vi "color2resistance.vi"() -> (5 "finish":bool, 6 "Correct or not":bool, 7 "Answear Time (sec)":dbl)   [LabVIEW 2014]
panel:
  out "Final Ans":dbl
  out "Band 3":u32(colorbox)=16750592
  out "Band 2":u32(colorbox)=16067327
  out "Band 1":u32(colorbox)=16776960
  in  "Resistor Colors":u32[](array[colorbox])=[0, 16730368, 16711680, 16750592, 16776960, 6618880, 3381759, 16067327, 11776947, 16448250]
  out "Question":dbl
  out "color 1":u32
  out "color 2":u32
  out "color 3":u32
  out "finish time":u32
  out "start time":u32
  out "Yout Answear":dbl
  in  "Enter":bool
  in  "Cluster":T1
  # "Please answear the resistance value corresponding to the color codes shown on the left"
  # "physical keyborad位置設計\n\nF1對應數字鍵1\nF2對應數字鍵2\nF3對應數字鍵3\nF4對應數字鍵4\nF5對應數字鍵5\nF6對應數字鍵6\nF7對應數字鍵7\nF8對應數字鍵8\nF9對應數字鍵9\nF10對應數字鍵0\nF11對符號 . \nDELETE對應Clear"
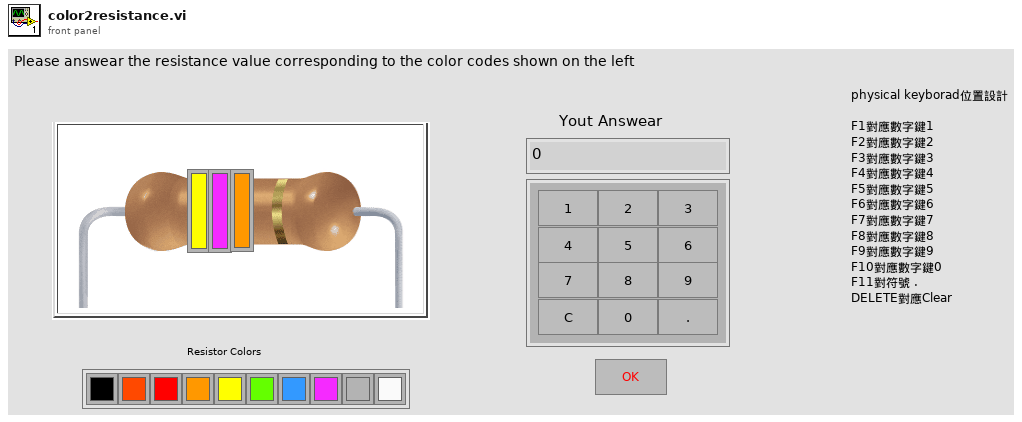
[diagram p1: front panel]
types:
  T1 = cluster{"1":bool, "2":bool, "3":bool, "4":bool, "5":bool, "6":bool, "7":bool, "8":bool, "9":bool, "0":bool, ".":bool, "C":bool}
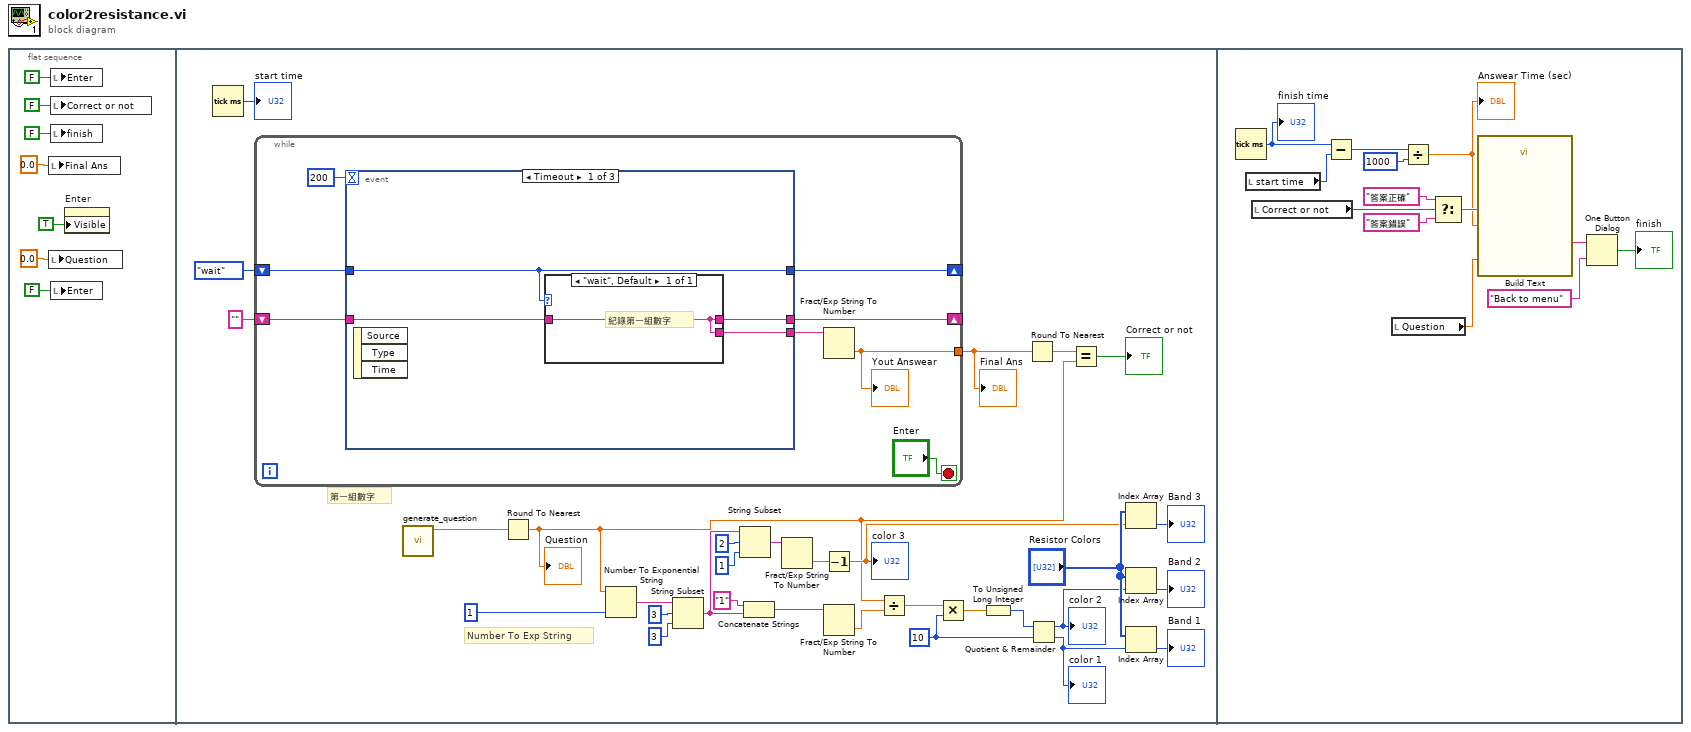
[diagram p0: block diagram]
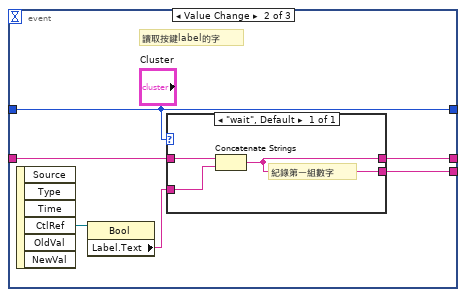
[diagram p2: hidden frame]
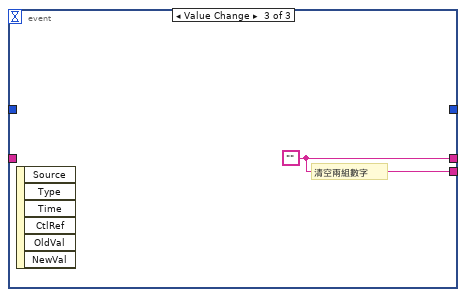
[diagram p3: hidden frame]
diagram:
  n1 = flat-sequence {
    frame #0 {
      n2 = local write "Final Ans"(0.0 ("Answear")) -> ()
      n3 = local write "Question"(0.0 ("Question")) -> ()
      n4 = local write "Enter"(FALSE ("stop")) -> ()
      n5 = local write "Correct or not"(FALSE ("Correct or not")) -> ()
      n6 = local write "finish"(FALSE ("finish")) -> ()
      n7 = local write "Enter"(FALSE ("Enter")) -> ()
      n8 = property on="Enter" class="Bool (strict)"("Visible"=TRUE) -> ()  [unwired: 2 in, 2 out]
    }
    frame #1 {
      w16 = u32 10 ("y")
      # "Number To Exp String"
      # "第一組數字"
      n9 = Tick Count (ms)() -> (millisecond timer value=→"start time":u32)
      n10 = while {
        shift-right: [w42] -> _
        shift-left: "" -> [w46]
        shift-right: [w44] -> _
        shift-left: enum16{"wait", "add", "sub", "mul", "div"}."wait" -> [w45]
        tunnel: [w39] -> w9
        stop <- "Enter" stop-if-true
        n11 = event shown="[0] Timeout" {
          selector: _ -> [_ _ _]
          dyn-events: _ -> [_ _ _]
          timeout: 200 -> [_ _ _]
          tunnel: w46 -> [w50 w57 _]
          tunnel: w45 -> [w47 w55 _]
          tunnel: [w47 w55 _] -> w44
          tunnel: [w49 w54 w61] -> w40
          tunnel: [w48 w53 w61] -> w42
          event Timeout {
            n12 = event-data() -> ()  [unwired: 1 in, 3 out]
            n13 = case shown="\"wait\", Default" w47 {
              tunnel: w50 -> [w51]
              tunnel: [w51] -> w49
              tunnel: [w51] -> w48
              frame "wait", Default {
                # "紀錄第一組數字"
              }
            }
          }
          event "Cluster..", "Cluster.1", "Cluster.2", "Cluster.3", "Cluster.4", "Cluster.5", "Cluster.6", "Cluster.7", "Cluster.9", "Cluster.8", "Cluster.0": Value Change {
            # "讀取按鍵label的字"
            n14 = event-data() -> ("CtlRef"=w56:refnum<vi>)  [unwired: 1 in, 5 out]
            n15 = property class="Bool"(reference=w56) -> ("Label.Text"=w52:string)  [unwired: 1 in, 2 out]
            n16 = case shown="\"wait\", Default" w55 {
              tunnel: w57 -> [w59]
              tunnel: [w58] -> w54
              tunnel: [w58] -> w53
              tunnel: w52 -> [w60]
              frame "wait", Default {
                # "紀錄第一組數字"
                n17 = Concatenate Strings(w59, w60) -> (w58:string)
              }
            }
          }
          event "Cluster.C": Value Change {
            w61 = ""
            # "清空兩組數字"
            n18 = event-data() -> ()  [unwired: 1 in, 6 out]
          }
        }
        n19 = Fract/Exp String To Number(string=w40) -> (number=w39:dbl)  [unwired: 3 in, 1 out]
        "Yout Answear" <- w39
      }
      "Final Ans" <- w9
      n20 = call "generate_question.vi"() -> ("Question"=w11:dbl)  [unwired: 11 in]
      n21 = Round To Nearest(number=w11) -> (nearest integer value=w10:dbl)
      "Question" <- w10
      n22 = Number To Exponential String(number=w10, precision (6)=i16 1) -> (E-format string=w34:string)  [unwired: 2 in]
      n23 = String Subset(string=w34, offset (0)=3, length (rest)=3 ("length (rest)")) -> (substring=w29:string)
      n24 = String Subset(string=w29, offset (0)=2, length (rest)=1 ("length (rest)")) -> (substring=w27:string)
      n25 = Concatenate Strings("1" ("string"), w29) -> (w31:string)
      n26 = Fract/Exp String To Number(string=w27) -> (number=w24:dbl)  [unwired: 3 in, 1 out]
      n27 = Decrement(x=w24) -> (x-1=w15:dbl)
      "color 3" <- w15
      n28 = Fract/Exp String To Number(string=w31) -> (number=w26:dbl)  [unwired: 3 in, 1 out]
      n29 = Divide(x=w10, y=w26) -> (x/y=w25:dbl)
      n30 = Multiply(x=w25, y=w16) -> (x*y=w23:dbl)
      n31 = To Unsigned Long Integer(number=w23) -> (unsigned 32bit integer=w22:u32)
      n32 = Round To Nearest(number=w9) -> (nearest integer value=w8:dbl)
      n33 = Quotient & Remainder(x=w22, y=w16) -> (x-y*floor(x/y)=w17:u32, floor(x/y)=w14:u32)
      "color 2" <- w17
      "color 1" <- w14
      n34 = Equal?(x=w8, y=w10) -> (x = y?=→"Correct or not":bool)
      n35 = Index Array(array="Resistor Colors", index=w15) -> (element=→"Band 3":u32)
      n36 = Index Array(array="Resistor Colors", index=w17) -> (element=→"Band 2":u32)
      n37 = Index Array(array="Resistor Colors", index=w14) -> (element=→"Band 1":u32)
    }
    frame #2 {
      n38 = Tick Count (ms)() -> (millisecond timer value=w74:u32)
      "finish time" <- w74
      n39 = local read "start time"() -> (w73:u32)
      n40 = local read "Correct or not"() -> (w68:bool)
      n41 = Subtract(x=w74, y=w73) -> (x-y=w72:u32)
      n42 = local read "Question"() -> (w62:dbl)
      n43 = Divide(x=w72, y=u32 1000) -> (x/y=w66:dbl)
      "Answear Time (sec)" <- w66
      n44 = Select(t="答案正確", s=w68, f="答案錯誤") -> (s? t:f=w67:string)
      n45 = call "Build Text"("correct_str"=w67, "ans_time"=w66, "question"=w62) -> ("Result"=w65:string)  [unwired: 11 in, 1 out]
      n46 = One Button Dialog(message=w65, button name ("OK")="Back to menu") -> (true=→"finish":bool)
    }
  }
